vi "T.vi"() -> ()   [LabVIEW 2018]
panel:
  out "Qx0":bool
  out "Qx1":bool
  in  "stop":bool
  out "Z0":bool
  out "Z1":bool
  in  "Y":bool
  in  "X":bool
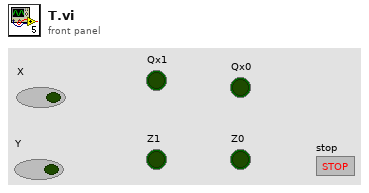
[diagram p1: front panel]
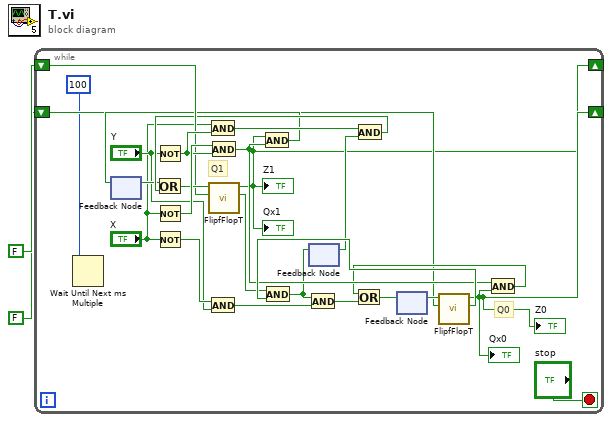
[diagram p0: block diagram]
diagram:
  n1 = while {
    shift-right: [w6] -> _
    shift-left: FALSE -> [w23]
    shift-right: [w7] -> _
    shift-left: FALSE -> [w10]
    stop <- "stop" stop-if-true
    # "Q1"
    # "Q0"
    n2 = Wait Until Next ms Multiple(millisecond multiple=u32 100) -> ()  [unwired: 1 out]
    n3 = feedback #1() -> (w18:bool)  [unwired: 1 in]
    n4 = Not(x="Y") -> (.not. x?=w27:bool)
    n5 = Not(x="X") -> (.not. x?=w28:bool)
    n6 = Not(x="X") -> (.not. x?=w16:bool)
    n7 = And(x="X", y=w27) -> (x .and. y?=w21:bool)
    n8 = And(x=w16, y="Y") -> (x .and. y?=w5:bool)
    n9 = And(x=w28, y=w27) -> (x .and. y?=w17:bool)
    n10 = feedback #2() -> (w20:bool)  [unwired: 1 in]
    n11 = And(x=w21, y=w20) -> (x .and. y?=w22:bool)
    n12 = Or(x=w18, y=w22) -> (x .or. y?=w24:bool)
    n13 = call "FlipfFlopT.vi"("Q"=w23, "T"=w24) -> ("QN*"=w25:bool, "Q*"=w6:bool)  [unwired: 8 in]
    "Z1" <- w6
    "Qx1" <- w6
    n14 = And(x=w6, y=w17) -> (x .and. y?=w19:bool)
    n15 = feedback-in #1(w19) -> ()
    n16 = feedback #3() -> (w11:bool)  [unwired: 1 in]
    n17 = call "FlipfFlopT.vi"("Q"=w10, "T"=w11) -> ("QN*"=w26:bool, "Q*"=w7:bool)  [unwired: 8 in]
    "Z0" <- w7
    "Qx0" <- w7
    n18 = And(x=w25, y=w26) -> (x .and. y?=w4:bool)
    n19 = And(x=w4, y=w5) -> (x .and. y?=w3:bool)
    n20 = feedback-in #2(w4) -> ()
    n21 = And(x=w17, y=w7) -> (x .and. y?=w13:bool)
    n22 = Or(x=w13, y=w3) -> (x .or. y?=w12:bool)
    n23 = feedback-in #3(w12) -> ()
  }
